vi "Read physical channels.vi"(8 "error in (no error)":errorcluster, 11 "Hardware Buzzer in":refnum<class "Hardware Buzzer.lvclass">) -> (0 "error out":errorcluster, 2 "physical channels":tag="Dev3/ai0:3", 3 "Hardware Buzzer out":refnum<class "Hardware Buzzer.lvclass">)   [LabVIEW 2024, in "Hardware Buzzer.lvlib" / "Hardware Buzzer.lvclass"]
uses:
  Hardware Buzzer.lvclass
  Hardware Buzzer.lvclass/Hardware Buzzer.ctl
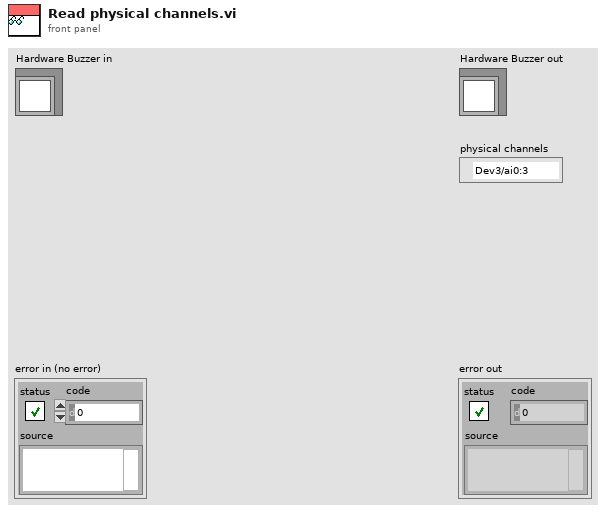
[diagram p1: front panel]
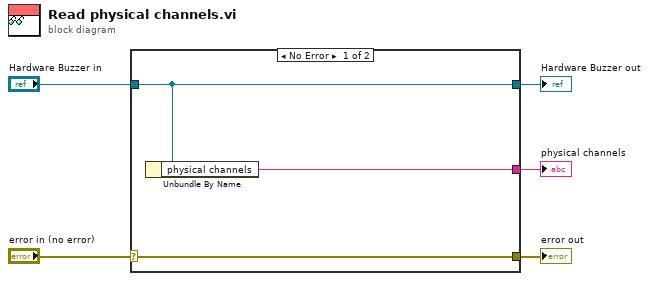
[diagram p0: block diagram]
diagram:
  n1 = case shown="No Error" "error in (no error)" {
    selector: "error in (no error)" -> [w8 w9]
    tunnel: [w8 w9] -> w4
    tunnel: [w7 w10] -> w2
    tunnel: "Hardware Buzzer in" -> [w7 w10]
    tunnel: [w6 _] -> w1
    frame No Error {
      n2 = Unbundle By Name(w7) -> ("physical channels"=w6:tag)
    }
    frame Error {
    }
  }
  "error out" <- w4
  "Hardware Buzzer out" <- w2
  "physical channels" <- w1
